vi "STOP.vi"(11 "Pump_1AI_1DO_2DI in":refnum<class "ValveModbus.lvclass">) -> (3 "Pump_1AI_1DO_2DI out":refnum<class "ValveModbus.lvclass">)   [LabVIEW 2019, in "ValveModbus.lvclass"]
uses:
  ValveModbus.lvclass
  ValveModbus.lvclass/ValveModbus.ctl
  TypeDef/StateValveModbus.ctl
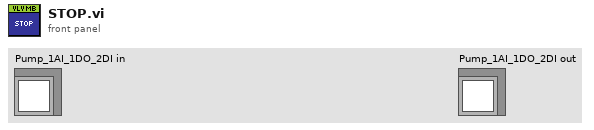
[diagram p1: front panel]
types:
  T1 = typedef "StateValveModbus.ctl" = enum16{"IDLE", "OPEN", "CLOSE", "OPENING", "CLOSING", "STOP"}
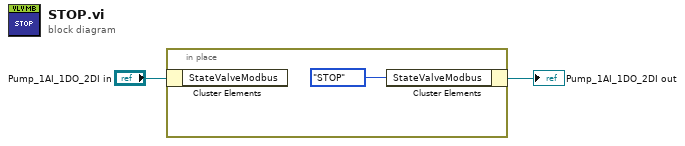
[diagram p0: block diagram]
diagram:
  n1 = in-place {
    n2 = in-place-cluster #1("Pump_1AI_1DO_2DI in") -> ()  [unwired: 1 out]
    n3 = in-place-cluster #1("StateValveModbus"=StateValveModbus."STOP") -> (→"Pump_1AI_1DO_2DI out":refnum<class "ValveModbus.lvclass">)
  }
